vi "setDataU8.vi"(0 "FixedFrameBuilder in":refnum<class "FixedFrameBuilder.lvclass">, 5 "Index":i32, 7 "Data":u8, 11 "error in (no error)":errorcluster) -> (4 "FixedFrameBuilder out":refnum<class "FixedFrameBuilder.lvclass">, 15 "error out":errorcluster)   [LabVIEW 2016, in "RTModbus.lvlib" / "FixedFrameBuilder.lvclass"]
uses:
  FixedFrameBuilder.lvclass
  FixedFrameBuilder.lvclass/FixedFrameBuilder.ctl
  Common_RT_Utilities/U8ArrayBuilderManualIndexing/U8ArrayBuilderManualIndexing.lvclass
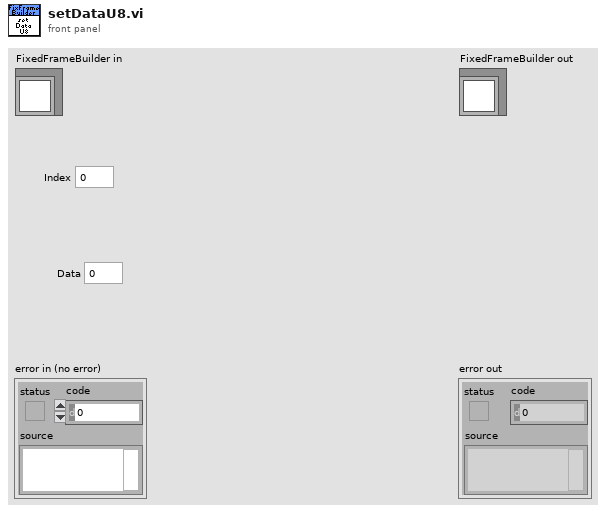
[diagram p1: front panel]
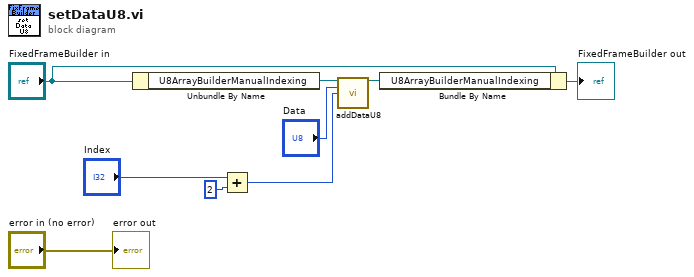
[diagram p0: block diagram]
diagram:
  n1 = Unbundle By Name("FixedFrameBuilder in") -> ("U8ArrayBuilderManualIndexing"=w4:refnum<class "U8ArrayBuilderManualIndexing.lvclass">)
  n2 = Add(x="Index", y=2) -> (x+y=w7:i32)
  n3 = call "addDataU8.vi"("U8ArrayBuilderManualIndexing in"=w4, "Data"="Data", "Index"=w7) -> ("U8ArrayBuilderManualIndexing out"=w5:refnum<class "U8ArrayBuilderManualIndexing.lvclass">)  [unwired: 10 in, 2 out]
  n4 = Bundle By Name(cluster="FixedFrameBuilder in", "U8ArrayBuilderManualIndexing"=w5) -> (→"FixedFrameBuilder out":refnum<class "FixedFrameBuilder.lvclass">)
  "error out" <- "error in (no error)"
